vi "getSequenceStepEnables.vi"(8 "error in":errorcluster, 10 "Slave Address (7-bit)":u8, 11 "I2C Ref In":T2) -> (0 "error out":errorcluster, 2 "enables":T1, 3 "I2C Ref Out":T2)   [LabVIEW 2018]
uses:
  <vilib>/myRIO/Instrument Drivers/Onboard IO/I2C/typedefs/I2C Reference.ctl
  <vilib>/myRIO/Common/Instrument Driver Framework/Utilities/typedefs/myRIO Generic Hardware Reference.ctl
  <vilib>/myRIO/Common/Instrument Driver Framework/Utilities/typedefs/Hardware Version Enum.ctl
  <vilib>/myRIO/Common/Instrument Driver Framework/Utilities/typedefs/myRIO v1.0 Reference.ctl
  <vilib>/myRIO/Common/Instrument Driver Framework/Utilities/typedefs/Generic FPGA Reference.ctl
  <vilib>/myRIO/Common/Instrument Driver Framework/myRIO v1.0/I2C/typedefs/I2C Channels Enum.ctl
  <vilib>/myRIO/Instrument Drivers/Onboard IO/I2C/typedefs/I2C Configuration.ctl
  <vilib>/myRIO/Instrument Drivers/Onboard IO/I2C/typedefs/I2C Transfer Rate.ctl
  <vilib>/Utility/error.llb/Error Cluster From Error Code.vi
  <vilib>/myRIO/Common/Instrument Driver Framework/myRIO v1.0/I2C/vis/myRIO v1.0 Write I2C.vi
  <vilib>/myRIO/Common/Instrument Driver Framework/myRIO v1.0/I2C/vis/myRIO v1.0 Read I2C.vi
  <vilib>/myRIO/Instrument Drivers/Onboard IO/I2C/I2C.lvlib
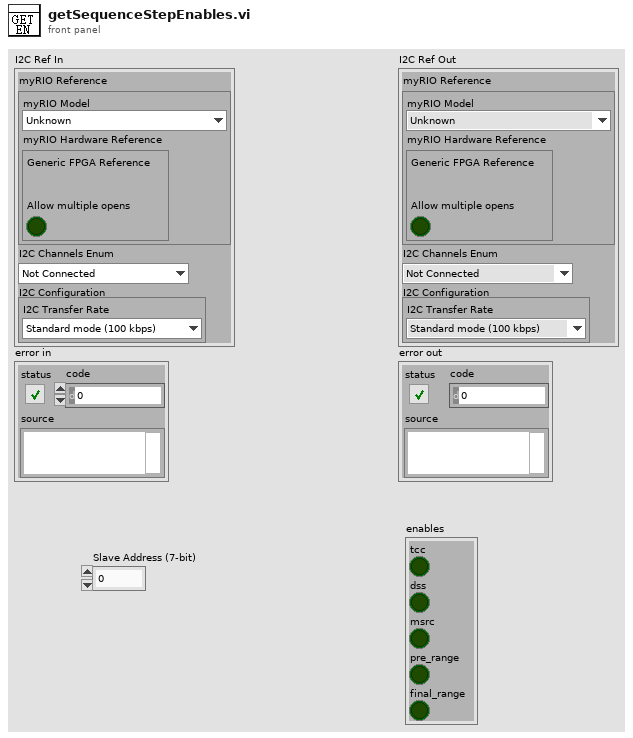
[diagram p1: front panel]
types:
  T1 = cluster{"tcc":bool, "dss":bool, "msrc":bool, "pre_range":bool, "final_range":bool}
  T2 = typedef "I2C.lvlib/I2C Reference.ctl" = cluster{"myRIO Reference":T3, "I2C Channels Enum":T7, "I2C Configuration":T8}
  T3 = typedef "myRIO Generic Hardware Reference.ctl" = cluster{"myRIO Model":T4, "myRIO Hardware Reference":T5}
  T4 = typedef "Hardware Version Enum.ctl" = enum16{"Unknown", "myRIO-1900", "myRIO-1950", "roboRIO", "NI ELVIS RIO CM", "ELVIS III"}
  T5 = typedef "myRIO v1.0 Reference.ctl" = cluster{"Generic FPGA Reference":T6, "Allow multiple opens":bool}
  T6 = typedef "Generic FPGA Reference.ctl" = refnum<k20>
  T7 = typedef "I2C Channels Enum.ctl" = enum16{"Not Connected", "A/I2C", "B/I2C", "I2C/I2C"}
  T8 = typedef "I2C.lvlib/I2C Configuration.ctl" = cluster{"I2C Transfer Rate":T9}
  T9 = typedef "I2C.lvlib/I2C Transfer Rate.ctl" = enum16{"Standard mode (100 kbps)", "Fast mode (400 kbps)"}
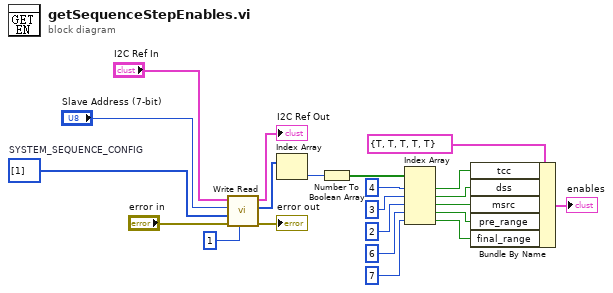
[diagram p0: block diagram]
diagram:
  w16 = u8[] [1]  # SYSTEM_SEQUENCE_CONFIG
  n1 = call <vilib>:"Write Read.vi"("Byte Count"=u32 1, "error in (no error)"="error in", "Bytes to Write"=w16, "Slave Address (7-bit)"="Slave Address (7-bit)", "I2C Ref In"="I2C Ref In") -> ("error out"=→"error out":errorcluster, "Bytes Read"=w15:u8[], "I2C Ref Out"=→"I2C Ref Out":T2)  [unwired: 3 in]
  n2 = Index Array(array=w15) -> (element=w14:u8)  [unwired: 1 in]
  n3 = Number To Boolean Array(number=w14) -> (Boolean array=w3:bool[])
  n4 = Index Array(array=w3, index #1=4, index #2=3, index #3=2, index #4=6, index #5=7) -> (element #1=w8:bool, element #2=w7:bool, element #3=w6:bool, element #4=w5:bool, element #5=w4:bool)
  n5 = Bundle By Name(cluster=T1 {"tcc"=TRUE, "dss"=TRUE, "msrc"=TRUE, "pre_range"=TRUE, "final_range"=TRUE}, "tcc"=w8, "dss"=w7, "msrc"=w6, "pre_range"=w5, "final_range"=w4) -> (→"enables":T1)
